vi "AppendObjectNameIfError.vi"(8 "error in (no error)":errorcluster, 10 "GObj Refnum":refnum<vi>, 11 "Object Layout in":refnum<class "Object Layout.lvclass">) -> (0 "error out":errorcluster, 3 "Object Layout out":refnum<class "Object Layout.lvclass">)   [LabVIEW 2010, in "NI_SE_Front Panel Layout.lvlib" / "Object Layout.lvclass"]
uses:
  Object Layout.lvclass
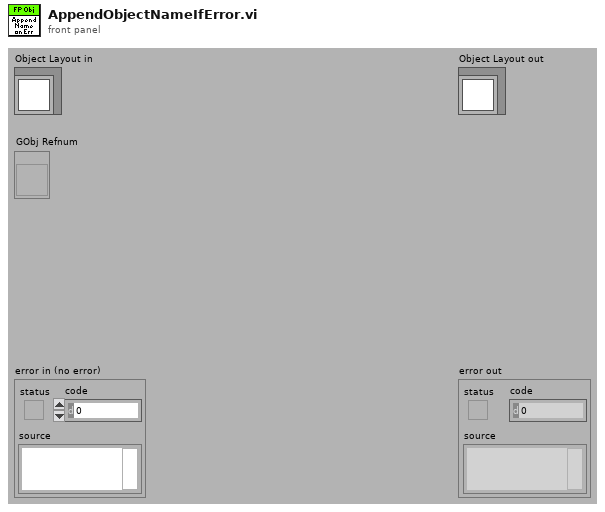
[diagram p1: front panel]
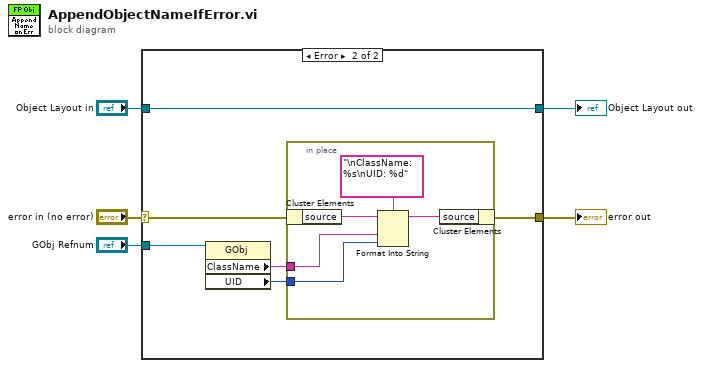
[diagram p0: block diagram]
diagram:
  n1 = case shown="Error" "error in (no error)" {
    selector: "error in (no error)" -> [w6 w11]
    tunnel: [w6 w10] -> w4
    tunnel: [w7 w13] -> w2
    tunnel: "Object Layout in" -> [w7 w13]
    tunnel: "GObj Refnum" -> [_ w12]
    frame No Error {
    }
    frame Error {
      n2 = property class="GObj"(reference=w12) -> ("ClassName"=w9:string, "UID"=w8:i32)  [unwired: 1 in, 2 out]
      n3 = in-place {
        in-place-border: w9 -> [w16]
        in-place-border: w8 -> [w14]
        n4 = in-place-cluster #1(w11) -> ("source"=w18:string)
        n5 = Format Into String(format string="\nClassName: %s\nUID: %d", initial string=w18, w16, w14) -> (resulting string=w17:string)  [unwired: 1 in, 1 out]
        n6 = in-place-cluster #1("source"=w17) -> (w10:errorcluster)
      }
    }
  }
  "error out" <- w4
  "Object Layout out" <- w2
